vi "get max or min by parabolic approx.vi"(0 "Array":dbl[](array[numeric]), 1 "max/min":bool=TRUE) -> (2 "y max":dbl=nan, 3 "x at max":dbl=nan)   [LabVIEW 2024]
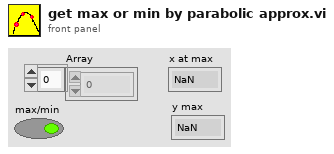
[diagram p1: front panel]
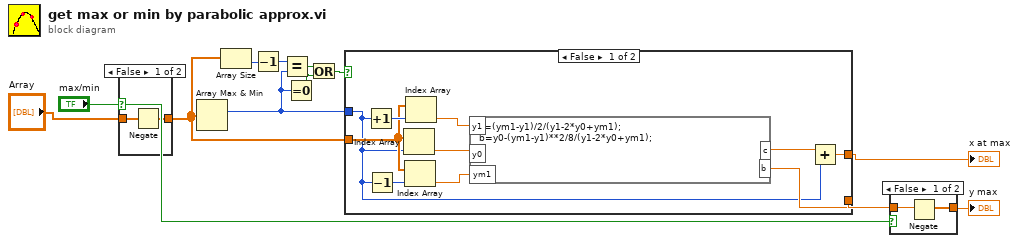
[diagram p0: block diagram]
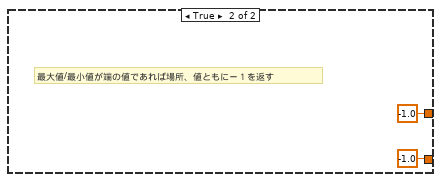
[diagram p2: hidden frame]
diagram:
  n1 = case shown="False" "max/min" {
    tunnel: "Array" -> [w14 w15]
    tunnel: [w13 w15] -> w7
    frame False {
      n2 = Negate(x=w14) -> (-x=w13:dbl[])
    }
    frame True {
    }
  }
  n3 = Array Max & Min(array=w7) -> (max index (indices)=w5:i32)  [unwired: 3 out]
  n4 = Array Size(array=w7) -> (size(s)=w6:i32)
  n5 = Decrement(x=w6) -> (x-1=w1:i32)
  n6 = Equal?(x=w1, y=w5) -> (x = y?=w4:bool)
  n7 = Equal To 0?(x=w5) -> (x = 0?=w3:bool)
  n8 = Or(x=w4, y=w3) -> (x .or. y?=w2:bool)
  n9 = case shown="False" w2 {
    tunnel: [w25 -1.0] -> w12
    tunnel: [w18 -1.0 ("b")] -> w8
    tunnel: w7 -> [w17 _]
    tunnel: w5 -> [w16 _]
    frame False {
      n10 = Increment(x=w16) -> (x+1=w19:i32)
      n11 = Decrement(x=w16) -> (x-1=w20:i32)
      n12 = Index Array(array=w17, index=w16) -> (element=w22:dbl)
      n13 = Index Array(array=w17, index=w20) -> (element=w23:dbl)
      n14 = Index Array(array=w17, index=w19) -> (element=w21:dbl)
      n15 = formula code="c=(ym1-y1)/2/(y1-2*y0+ym1);\nb=y0-(ym1-y1)**2/8/(y1-2*y0+ym1);"("ym1"=w23, "y0"=w22, "y1"=w21) -> ("c"=w24:dbl, "b"=w18:dbl)
      n16 = Add(x=w24, y=w16) -> (x+y=w25:dbl)
    }
    frame True {
      # "最大値/最小値が端の値であれば場所、値ともにー１を返す"
    }
  }
  "x at max" <- w12
  n17 = case shown="False" "max/min" {
    tunnel: [w28 w30] -> w9
    tunnel: w8 -> [w29 w30]
    frame False {
      n18 = Negate(x=w29) -> (-x=w28:dbl)
    }
    frame True {
    }
  }
  "y max" <- w9
